vi "AD5933_GetAllRegVal (NI-845x I2C)(SubVI).vi"(8 "error in (no error)":errorcluster, 11 "NI-845x Config for I2C (out) in":T3) -> (0 "error out":errorcluster, 2 "read data":u8[](array[numeric]), 3 "NI-845x Config for I2C (out) out":T3)   [LabVIEW 2017]
uses:
  <vilib>/ni845x/ni845x.llb/ni845xI2cConfiguration.ctl
  <vilib>/ni845x/ni845x.llb/ni845xControl.ctl
  TypeDefs/AD5933_CommandCodes.ctl
  TypeDefs/AD5933_Registers.ctl
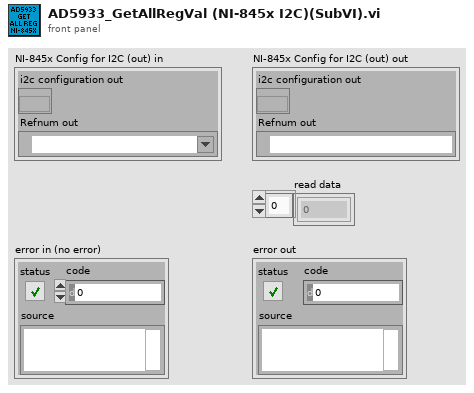
[diagram p1: front panel]
types:
  T1 = typedef "ni845xI2cConfiguration.ctl" = refnum<k20>
  T2 = typedef "ni845xControl.ctl" = refnum<k21>
  T3 = cluster{"i2c configuration out":T1, "Refnum out":T2}
  T4 = typedef "AD5933_CommandCodes.ctl" = u8
  T5 = typedef "AD5933_Registers.ctl" = u8
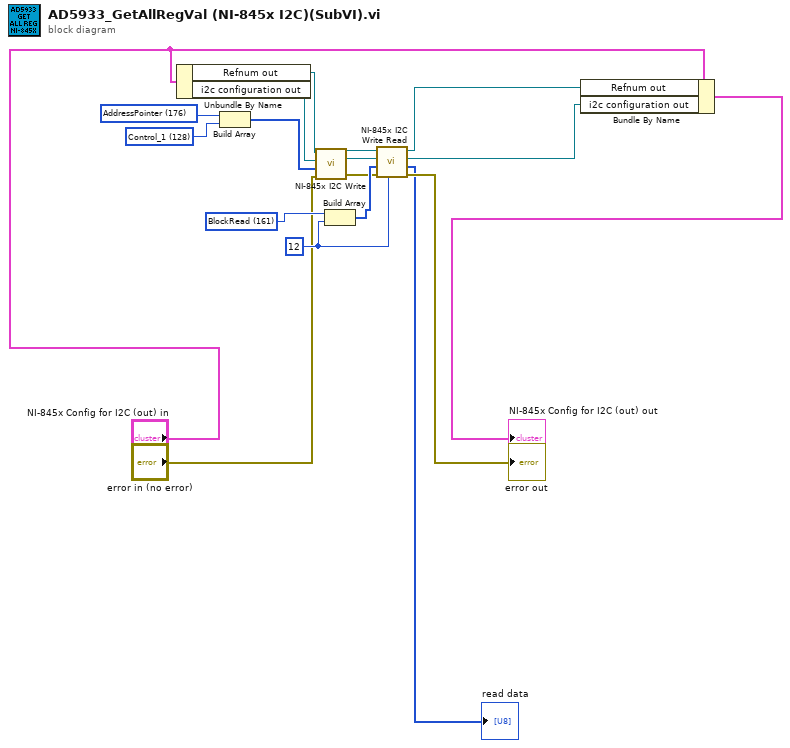
[diagram p0: block diagram]
diagram:
  w18 = 12
  w16 = T4 161 items=["BlockWrite"=160, "BlockRead"=161, "AddressPointer"=176] ("CommandCodes")
  w4 = T5 128 items=["Control_1"=128, "Control_0"=129, "StartFeq_2"=130, "StartFeq_1"=131, "StartFeq_0"=132, "FreqInc_2"=133, "FreqInc_1"=134, "FreqInc_0"=135, "NumOfInc_1"=136, "NumOfInc_0"=137, "NumOfSetCycl_1"=138, "NumOfSetCycl_0"=139, "Status"=143, "TempData_1"=146, "TempData_0"=147, "RealData_1"=148, "RealData_0"=149, "ImagData_1"=150, "ImagData_0"=151] ("Register")
  w5 = T4 176 items=["BlockWrite"=160, "BlockRead"=161, "AddressPointer"=176] ("CommandCodes")
  n1 = Unbundle By Name("NI-845x Config for I2C (out) in") -> ("Refnum out"=w6:T2, "i2c configuration out"=w7:T1)
  n2 = Build Array(w5, w4) -> (w11:T5[])
  n3 = call <vilib>:"NI-845x I2C Write.vi"("error in (no error)"="error in (no error)", "write data"=w11, "i2c configuration in"=w7, "device reference in"=w6) -> ("error out"=w10:errorcluster, "i2c configuration out"=w9:T1, "device reference out"=w8:T2)  [unwired: 5 in]
  n4 = Build Array(w16, w18) -> (w17:i32[])
  n5 = call <vilib>:"NI-845x I2C Write Read.vi"("num bytes to read"=w18, "error in (no error)"=w10, "write data"=w17, "i2c configuration in"=w9, "device reference in"=w8) -> ("error out"=→"error out":errorcluster, "read data"=→"read data":u8[], "i2c configuration out"=w2:T1, "device reference out"=w3:T2)  [unwired: 3 in]
  n6 = Bundle By Name(cluster="NI-845x Config for I2C (out) in", "Refnum out"=w3, "i2c configuration out"=w2) -> (→"NI-845x Config for I2C (out) out":T3)
